vi "Create.vi"(8 "error in (no error)":errorcluster, 10 "Size":T1) -> (0 "error out":errorcluster, 3 "Board out":refnum<class "Board.lvclass">)   [LabVIEW 2015, in "TronviewGame.lvlib" / "Board.lvclass"]
uses:
  Board.lvclass
  BoardSize.ctl
  Board.lvclass/Board.ctl
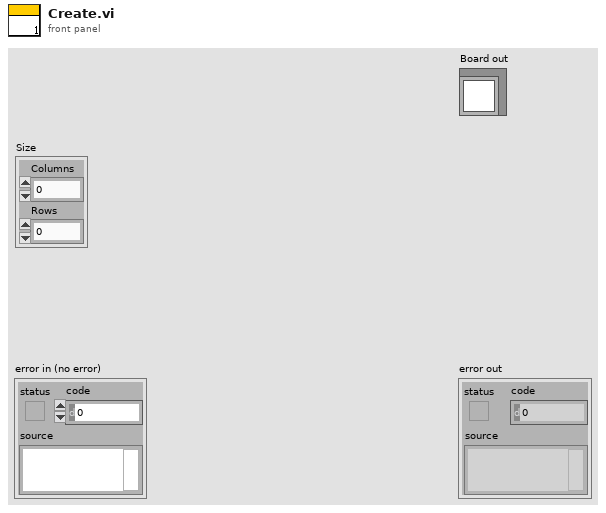
[diagram p1: front panel]
types:
  T1 = typedef "TronviewGame.lvlib/Board.lvclass/BoardSize.ctl" = cluster{"Columns":u32, "Rows":u32}
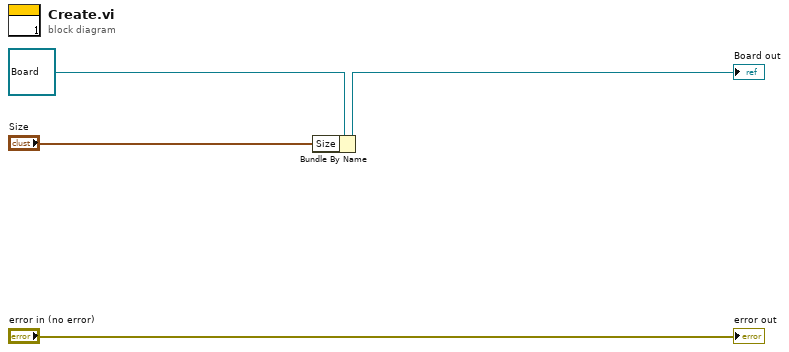
[diagram p0: block diagram]
diagram:
  n1 = Bundle By Name(cluster=refnum<class "Board.lvclass"> refnum ("Board in"), "Size"="Size") -> (→"Board out":refnum<class "Board.lvclass">)
  "error out" <- "error in (no error)"
